vi "Vector Mover.vi"(4 "Absolute/Relative (F/T)":bool, 5 "Movement Vector":dbl[](array[numeric])=[0.0, 0.0, 0.0, 0.0, 0.0], 6 "error in (no error)":errorcluster, 7 "Angular Speed":dbl, 8 "Vector Speed":dbl, 9 "controller in":refnum<k24>) -> (0 "error out":errorcluster={"status"=TRUE, "code"=-536337543, "source"="AerVectorMove: ERROR: F-word (LinearFeedRate) is zero"}, 3 "controller out":refnum<k24>)   [LabVIEW 2011]
uses:
  C:/Users/Admin/Desktop/Gantry Code Transfer/source/Code Transfer/Aerotech.A3200.dll
  Aerotech.A3200.dll
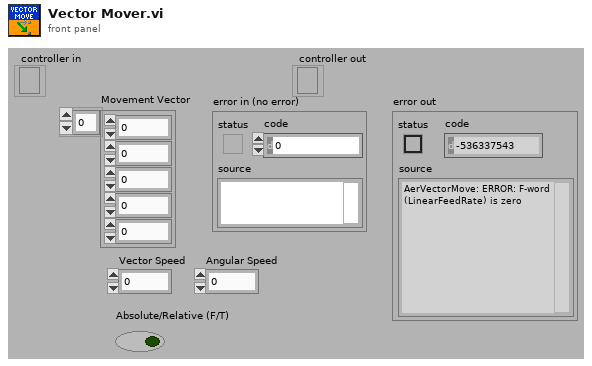
[diagram p1: front panel]
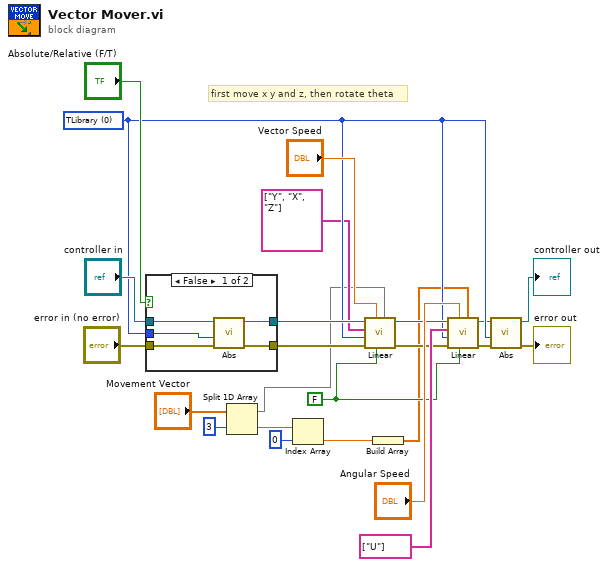
[diagram p0: block diagram]
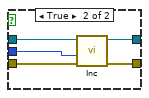
[diagram p2: hidden frame]
diagram:
  w11 = FALSE ("return immediately")
  w14 = 0 items=["TLibrary", "T01", "T02", "T03", "T04", "T05", "T06", "T07", "T08", "T09", "T10", "T11", "T12", "T13", "T14", "T15", "T16", "T17", "T18", "T19", "T20", "T21", "T22", "T23", "T24", "T25", "T26", "T27", "T28", "T29", "T30", "T31"] ("taskId")
  # "first move x y and z, then rotate theta"
  n1 = case shown="False" "Absolute/Relative (F/T)" {
    tunnel: w14 -> [w29 w34]
    tunnel: "controller in" -> [w28 w33]
    tunnel: "error in (no error)" -> [w27 w30]
    tunnel: [w26 w31] -> w20
    tunnel: [w25 w32] -> w21
    frame False {
      n2 = call "Abs.vi"("error in (no error)"=w27, "taskId"=w29, "controller in"=w28) -> ("error out"=w26:errorcluster, "controller out"=w25:refnum<k24>)  [unwired: 7 in]
    }
    frame True {
      n3 = call "Inc.vi"("error in (no error)"=w30, "taskId"=w34, "controller in"=w33) -> ("error out"=w31:errorcluster, "controller out"=w32:refnum<k24>)  [unwired: 7 in]
    }
  }
  n4 = Split 1D Array(array="Movement Vector", index=3) -> (first subarray=w7:dbl[], second subarray=w1:dbl[])
  n5 = Index Array(array=w1, index=0) -> (element=w4:dbl)
  n6 = call "Linear.vi"("distances"=w7, "return immediately"=w11, "speed"="Vector Speed", "error in (no error)"=w20, "taskId"=w14, "axis names"=string[] ["Y", "X", "Z"], "controller in"=w21) -> ("error out"=w16:errorcluster, "controller out"=w17:refnum<k24>)  [unwired: 3 in]
  n7 = Build Array(w4) -> (w5:dbl[])
  n8 = call "Linear.vi"("distances"=w5, "return immediately"=w11, "speed"="Angular Speed", "error in (no error)"=w16, "taskId"=w14, "axis names"=string[] ["U"], "controller in"=w17) -> ("error out"=w2:errorcluster, "controller out"=w3:refnum<k24>)  [unwired: 3 in]
  n9 = call "Abs.vi"("error in (no error)"=w2, "taskId"=w14, "controller in"=w3) -> ("error out"=→"error out":errorcluster, "controller out"=→"controller out":refnum<k24>)  [unwired: 7 in]
